vi "IPI_Cal_Point TO Line.vi"(0 "Image in":T1(plugin-control), 1 "Point1 (Pixels) First":cluster{"X":sgl, "Y":sgl}, 2 "Point1 (Pixels) Second":cluster{"X":sgl, "Y":sgl}, 5 "Start Point":cluster{"X":i32, "Y":i32}) -> (14 "Image Out":T1(plugin-control), 17 "Piex":string, 18 "Dist piex":dbl, 19 "error out":errorcluster)   [LabVIEW 2015]
uses:
  <vilib>/Analysis/NI_AALPro.lvlib
panel:
  in  "error in (no error)":errorcluster
  out "result":string
  out "y 焦点":dbl
  out "X 焦点":dbl
  out "b2":dbl
  out "k2":dbl
  out "b1":dbl caption="截距"
  out "k1":dbl caption="斜率"
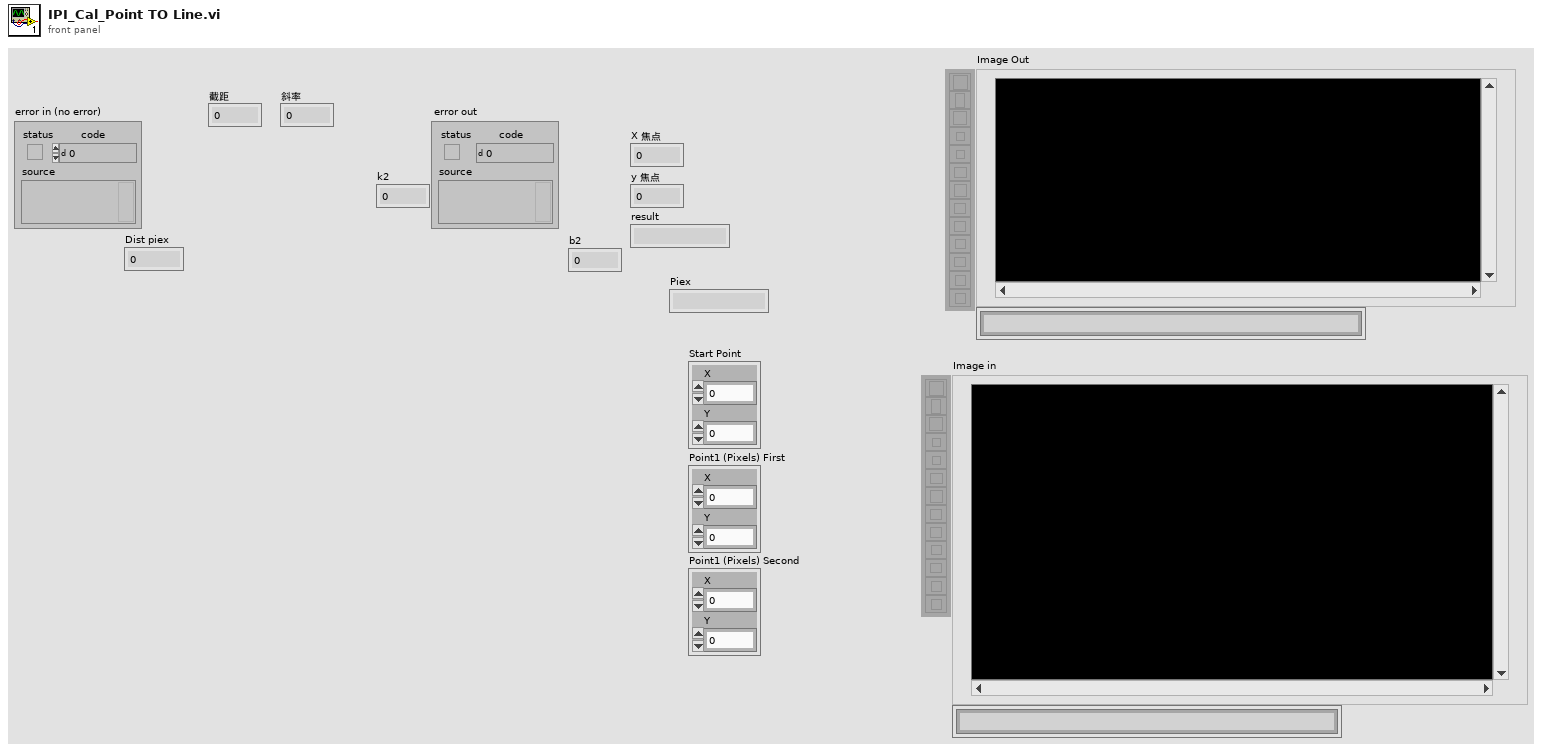
[diagram p1: front panel]
types:
  T1 = typedef "IMAQ Image.ctl" = refnum<image>
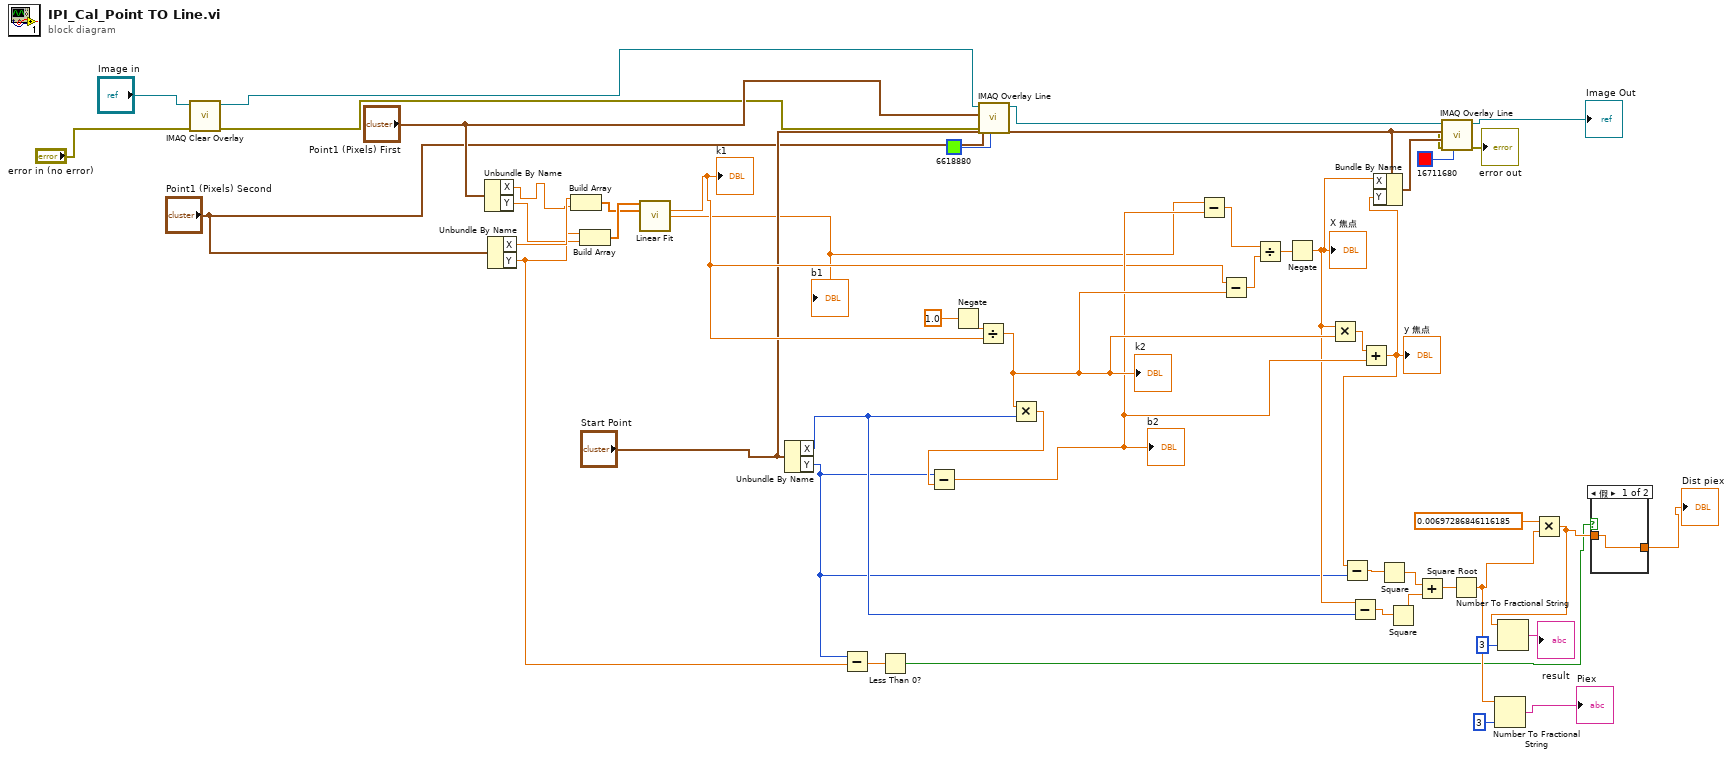
[diagram p0: block diagram]
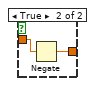
[diagram p2: hidden frame]
diagram:
  n1 = call "IMAQ Clear Overlay"("error in (no error)"="error in (no error)", "Image"="Image in") -> ("error out"=w7:errorcluster, "Image Out"=w9:T1)  [unwired: 8 in]
  n2 = Unbundle By Name("Point1 (Pixels) First") -> ("X"=w23:sgl, "Y"=w22:sgl)
  n3 = Unbundle By Name("Point1 (Pixels) Second") -> ("X"=w24:sgl, "Y"=w5:sgl)
  n4 = Build Array(w24, w23) -> (w49:sgl[])
  n5 = Build Array(w5, w22) -> (w50:sgl[])
  n6 = call <vilib>:"Linear Fit.vi"("Y"=w50, "X"=w49) -> ("slope"=w21:dbl, "intercept"=w16:dbl)  [unwired: 9 in, 3 out]
  "k1" <- w21
  "b1" <- w16
  n7 = Unbundle By Name("Start Point") -> ("X"=w31:i32, "Y"=w6:i32)
  n8 = Subtract(x=w6, y=w5) -> (x-y=w4:sgl)
  n9 = Less Than 0?(x=w4) -> (x < 0?=w2:bool)
  n10 = Negate(x=1.0) -> (-x=w46:dbl)
  n11 = Divide(x=w46, y=w21) -> (x/y=w41:dbl)
  "k2" <- w41
  n12 = call "IMAQ Overlay Line"("Color"=u32 6618880, "error in (no error)"=w7, "End Point"="Point1 (Pixels) Second", "Start Point"="Point1 (Pixels) First", "Image"=w9) -> ("error out"=w13:errorcluster, "Image Out"=w38:T1)  [unwired: 5 in]
  n13 = Multiply(x=w41, y=w31) -> (x*y=w45:dbl)
  n14 = Subtract(x=w6, y=w45) -> (x-y=w39:dbl)
  "b2" <- w39
  n15 = Subtract(x=w16, y=w39) -> (x-y=w44:dbl)
  n16 = Subtract(x=w21, y=w41) -> (x-y=w43:dbl)
  n17 = Divide(x=w44, y=w43) -> (x/y=w42:dbl)
  n18 = Negate(x=w42) -> (-x=w32:dbl)
  "X 焦点" <- w32
  n19 = Multiply(x=w32, y=w41) -> (x*y=w40:dbl)
  n20 = Subtract(x=w32, y=w31) -> (x-y=w30:dbl)
  n21 = Add(x=w40, y=w39) -> (x+y=w34:dbl)
  "y 焦点" <- w34
  n22 = Subtract(x=w34, y=w6) -> (x-y=w33:dbl)
  n23 = Bundle By Name(cluster="Start Point", "X"=w32, "Y"=w34) -> (w37:cluster{"X":i32, "Y":i32})
  n24 = Square(x=w33) -> (x^2=w29:dbl)
  n25 = Square(x=w30) -> (x^2=w28:dbl)
  n26 = Add(x=w29, y=w28) -> (x+y=w27:dbl)
  n27 = call "IMAQ Overlay Line"("Color"=u32 16711680, "error in (no error)"=w13, "End Point"=w37, "Start Point"="Start Point", "Image"=w38) -> ("error out"=→"error out":errorcluster, "Image Out"=→"Image Out":T1)  [unwired: 5 in]
  n28 = Square Root(x=w27) -> (sqrt(x)=w19:dbl)
  n29 = Number To Fractional String(number=w19, precision (6)=i16 3 ("精度(6)")) -> (F-format string=→"Piex":string)  [unwired: 2 in]
  n30 = Multiply(x=0.00697286846116185, y=w19) -> (x*y=w3:dbl)
  n31 = Number To Fractional String(number=w3, precision (6)=i16 3 ("精度(6)")) -> (F-format string=→"result":string)  [unwired: 2 in]
  n32 = case shown="假" w2 {
    tunnel: w3 -> [w51 w53]
    tunnel: [w51 w52] -> w1
    frame False {
    }
    frame True {
      n33 = Negate(x=w53) -> (-x=w52:dbl)
    }
  }
  "Dist piex" <- w1
